vi "onStart.vi"(8 "error in (no error)":errorcluster, 11 "Instrument.DAQ":refnum<class "Instrument.DAQ.lvclass">) -> (0 "error out":errorcluster, 3 "Instrument.DAQ out":refnum<class "Instrument.DAQ.lvclass">)   [LabVIEW 2019, in "Instrument.Lockin.lvlib" / "Instrument.DAQ.lvclass"]
uses:
  Instrument.DAQ.lvclass
  C:/Program Files/National Instruments/LabVIEW 2019/vi.lib/JKI/JKI SMO/SMO/SMO.lvclass
  Instrument.DAQ.lvclass/Instrument.DAQ.ctl
  <vilib>/JKI/JKI SMO/SMO/SMO.lvclass
panel:
  out "Generator Found?":bool
  out "DAQmx Found?":bool
  # "For instructions on how to use the JKI State Machine Objects, examples and video tutorials, visit:\nhttp://jki.net/state-machine-objects/\n\nJKI State Machine Objects™\nhttp://jki.net/state-machine-objects/\nCopyright (C) 2005-2015, JKI <info@jki.net>\nALL RIGHTS RESERVED"
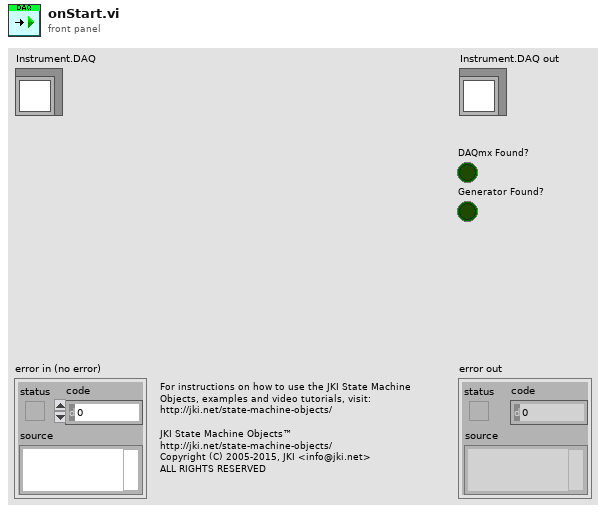
[diagram p1: front panel]
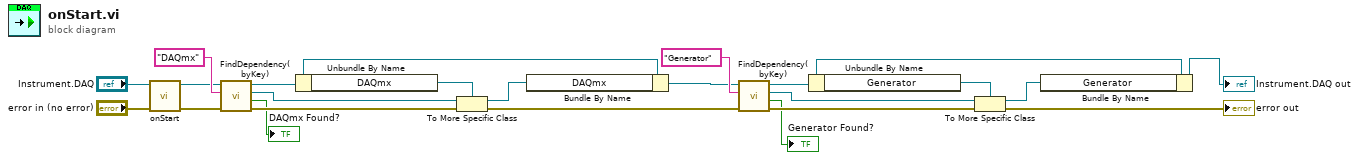
[diagram p0: block diagram]
diagram:
  n1 = call-parent "onStart.vi"("error in (no error)"="error in (no error)", "SMO"="Instrument.DAQ") -> ("error out"=w15:errorcluster, "SMO out"=w18:refnum<class "Instrument.DAQ.lvclass">)  [unwired: 8 in]
  n2 = call <vilib>:"FindDependency(byKey).vi"("error in (no error)"=w15, "Key"="DAQmx", "SMO in"=w18) -> ("error out"=w14:errorcluster, "Found?"=→"DAQmx Found?":bool, "Dependency"=w20:refnum<class "SMO.lvclass">, "SMO dup"=w13:refnum<class "Instrument.DAQ.lvclass">)  [unwired: 5 in]
  n3 = Unbundle By Name(w13) -> ("DAQmx"=w16:refnum<class "DAQmx.lvclass">)
  n4 = To More Specific Class(target class=w16, reference=w20, error in=w14) -> (specific class reference=w17:refnum<class "DAQmx.lvclass">, error out=w6:errorcluster)
  n5 = Bundle By Name(cluster=w13, "DAQmx"=w17) -> (w7:refnum<class "Instrument.DAQ.lvclass">)
  n6 = call <vilib>:"FindDependency(byKey).vi"("error in (no error)"=w6, "Key"="Generator", "SMO in"=w7) -> ("error out"=w12:errorcluster, "Found?"=→"Generator Found?":bool, "Dependency"=w8:refnum<class "SMO.lvclass">, "SMO dup"=w5:refnum<class "Instrument.DAQ.lvclass">)  [unwired: 5 in]
  n7 = Unbundle By Name(w5) -> ("Generator"=w11:refnum<class "Generator.lvclass">)
  n8 = To More Specific Class(target class=w11, reference=w8, error in=w12) -> (specific class reference=w10:refnum<class "Generator.lvclass">, error out=→"error out":errorcluster)
  n9 = Bundle By Name(cluster=w5, "Generator"=w10) -> (→"Instrument.DAQ out":refnum<class "Instrument.DAQ.lvclass">)
